vi "Handle M21.vi"(0 "reference in":refnum<class "PM_Group.lvclass">, 11 "error in (no error)":errorcluster) -> (4 "reference out":refnum<class "PM_Group.lvclass">, 15 "error out":errorcluster)   [LabVIEW 2019, in "PM_Group.lvclass"]
uses:
  PM_Group.lvclass
  C:/Users/ANENKOV_V1/Desktop/src/Device_class/Device.lvclass
  PM_Group.lvclass/PM_Group.ctl
  FPGA/TypeDef/AI index.ctl
  TypeDef/State Engine.ctl
  Device_class/Device.lvclass/Device.ctl
  Engine_1DO_2DI_class/Engine_1DO_2DI.lvclass/Engine_1DO_2DI.ctl
  FPGA/TypeDef/DO index.ctl
  AI_class/AI.lvclass/AI.ctl
  AnalogComparator_class/AnalogComparator.lvclass/AnalogComparator.ctl
  AnalogComparator_class/GetStatus.vi
  Engine_1DO_2DI_class/Engine_1DO_2DI.lvclass
  FPGA_API_class/FPGA API.lvclass
  AI_class/AI.lvclass
  Device_class/Device.lvclass
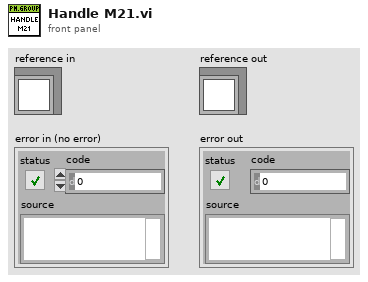
[diagram p1: front panel]
types:
  T1 = typedef "State Engine.ctl" = enum16{"Unknown", "Off", "TupningOn", "On", "TurningOff"}
  T2 = typedef "AI index.ctl" = u8
  T3 = typedef "DO index.ctl" = u8
  T4 = typedef "AI_Data.ctl" = cluster{"Stat Data":T5, "OutOfRangeMax":bool, "OutOfRangeMin":bool, "HIHI":bool, "HI":bool, "LO":bool, "LOLO":bool}
  T5 = typedef "AI Statistics Data.ctl" = cluster{"raw mean":dbl, "scl mean":dbl, "raw mean 1Hz":dbl, "scl mean 1Hz":dbl}
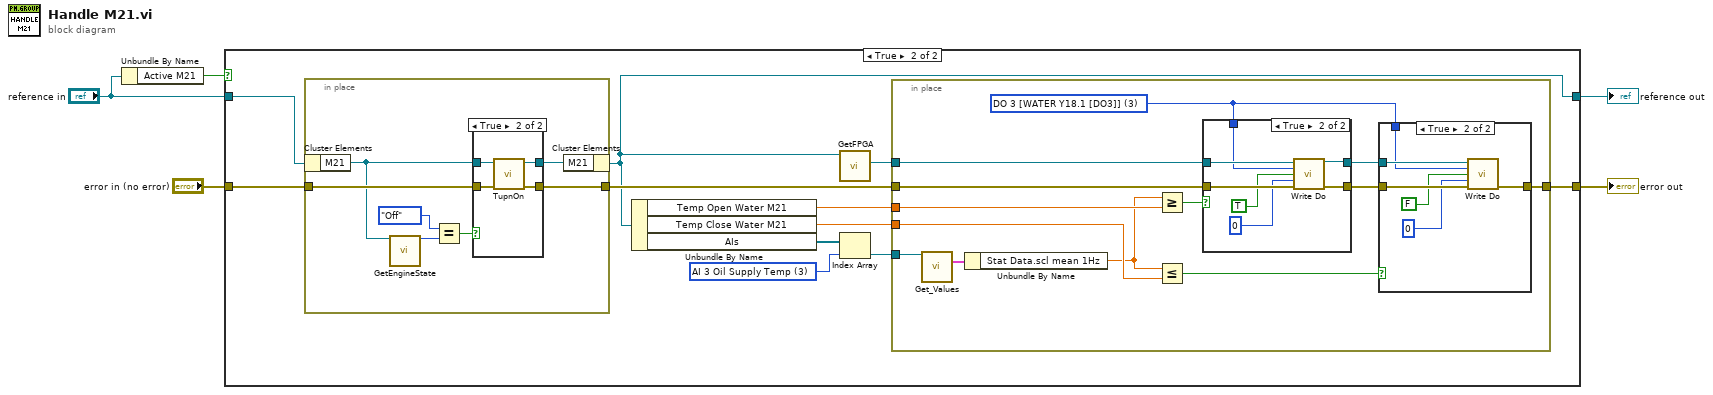
[diagram p0: block diagram]
diagram:
  n1 = Unbundle By Name("reference in") -> ("Active M21"=w1:bool)
  n2 = case shown="True" w1 {
    tunnel: "error in (no error)" -> [w6 w18]
    tunnel: "reference in" -> [w7 w17]
    tunnel: [w7 w9] -> w4
    tunnel: [w6 w8] -> w3
    frame False {
    }
    frame True {
      w15 = T2 3 items=["AI 0 Cooling Pump Level", "AI 1 Cooling Pump Temp", "AI 2 Oil Supply Level", "AI 3 Oil Supply Temp", "AI 4 ", "AI 5 Pressure Haskel", "AI 6 Pressure DUT", "AI 7 Pressure Chamber", "AI 8 Pressure Air inlet", "AI 9 Pressure Air outlet", "AI 10 Pressure Messure Line"] ("AI index")
      n3 = in-place {
        in-place-border: w18 -> [w52]
        in-place-border: [w50] -> w10
        n4 = in-place-cluster #1(w17) -> ("M21"=w51:refnum<class "Engine_1DO_2DI.lvclass">)
        n5 = call "GetEngineState.vi"("Engine"=w51) -> ("EngineState"=w53:T1)  [unwired: 10 in, 4 out]
        n6 = Equal?(x=State_Engine."Off" ("y"), y=w53) -> (x = y?=w49:bool)
        n7 = case shown="True" w49 {
          tunnel: w52 -> [w55 w60]
          tunnel: w51 -> [w56 w59]
          tunnel: [w56 w58] -> w48
          tunnel: [w55 w57] -> w50
          frame False {
          }
          frame True {
            n8 = call "TupnOn.vi"("error in (no error)"=w60, "Pump_1AI_1DO_2DI in"=w59) -> ("error out"=w57:errorcluster, "Pump_1AI_1DO_2DI out"=w58:refnum<class "Engine_1DO_2DI.lvclass">)  [unwired: 8 in]
          }
        }
        n9 = in-place-cluster #1("M21"=w48) -> (w9:refnum<class "PM_Group.lvclass">)
      }
      n10 = Unbundle By Name(w9) -> ("Temp Open Water M21"=w12:dbl, "Temp Close Water M21"=w13:dbl, "AIs"=w14:refnum<class "AI.lvclass">[])
      n11 = call "GetFPGA.vi"("Device in"=w9) -> ("FPGA API.lvclass"=w11:refnum<class "FPGA API.lvclass">)  [unwired: 10 in]
      n12 = Index Array(array=w14, index=w15) -> (element=w16:refnum<class "AI.lvclass">)
      n13 = in-place {
        in-place-border: w12 -> [w23]
        in-place-border: w13 -> [w24]
        in-place-border: w16 -> [w31]
        in-place-border: w10 -> [w29]
        in-place-border: [w26] -> w8
        in-place-border: w11 -> [w19]
        w20 = T3 3 items=["DO 0 [KP1 [DO 0]]", "DO 1 [ON KP2 [DO 1]]", "DO 2 [ON KP3 [DO 2]]", "DO 3 [WATER Y18.1 [DO3]]", "DO 4 [WATER Y18.2 [DO4]]", "DO 5 [KP6 Y29.1 33.7]", "DO 6 [KP7 Y29.2 33.8]", "DO 7 [KP8 Y29.3 33.9]", "DO 8 [KP9 Y29.4  33.12]", "DO 9 [KP10 Y29.5 33.1]", "DO 10 [KP11 Y29.6 33.2]", "DO 11 [KP12 Y29.7  33.13]", "DO 12 [KP13 Y29.8  33.11]", "DO 13 [KP14 Y29.9 33.10]", "DO 14 [KP15 Y29.10  33.6]", "DO 15 [KP16 Y29.11  33.5]", "DO 16 [KP17 Y29.12  33.4]", "DO 17 [KP18 Y29.13 33.3]", "DO 18 [AIR KP19]", "DO 19 [STEP DRIVE EN KP20]", "DO 20 [KP21 Y44.1 OPEN]", "DO 21 [ KP22 Y44.1 CLOSE]", "DO 22 [ KP23 Y44.2 OPEN]", "DO 23", "DO 24 [STEP DRIVE 1]", "DO 25 [STEP DRIVE 2]"] ("#DO")
        n14 = call "Get_Values.vi"("reference in"=w31) -> ("Data"=w30:T4)  [unwired: 14 in]
        n15 = Unbundle By Name(w30) -> ("Stat Data.scl mean 1Hz"=w21:dbl)
        n16 = Greater Or Equal?(x=w21, y=w23) -> (x >= y?=w28:bool)
        n17 = Less Or Equal?(x=w21, y=w24) -> (x <= y?=w22:bool)
        n18 = case shown="True" w28 {
          tunnel: w29 -> [w39 w45]
          tunnel: w19 -> [w40 w47]
          tunnel: [w40 w46] -> w25
          tunnel: [w39 w44] -> w27
          tunnel: w20 -> [_ w42]
          frame False {
          }
          frame True {
            n19 = call-dynamic "Write Do.vi"("FPGA API in"=w47, "#DO"=w42, "value"=TRUE, "Time uSec"=u32 0, "error in (no error)"=w45) -> ("FPGA API out"=w46:refnum<class "FPGA API.lvclass">, "error out"=w44:errorcluster)  [unwired: 9 in]
          }
        }
        n20 = case shown="True" w22 {
          tunnel: w25 -> [_ w38]
          tunnel: w27 -> [w32 w37]
          tunnel: [w32 w36] -> w26
          tunnel: w20 -> [_ w35]
          frame False {
          }
          frame True {
            n21 = call-dynamic "Write Do.vi"("FPGA API in"=w38, "#DO"=w35, "value"=FALSE, "Time uSec"=u32 0, "error in (no error)"=w37) -> ("error out"=w36:errorcluster)  [unwired: 9 in, 1 out]
          }
        }
      }
    }
  }
  "reference out" <- w4
  "error out" <- w3
